vi "Access DB Path.vi"(9 "Password":string, 10 "ping":bool, 11 "database":string="database1.mdb") -> (2 "Connection information":string, 3 "Path out":string)   [LabVIEW 2016, in "Access Lib.lvlib"]
uses:
  Access Lib.lvlib
  <vilib>/Utility/sysdir.llb/System Directory Type.ctl
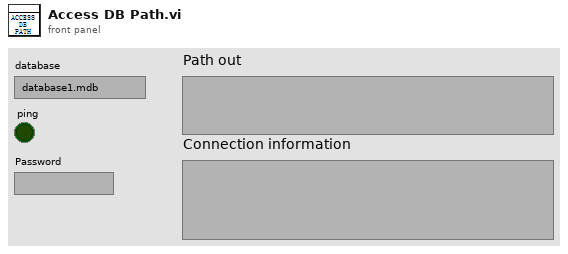
[diagram p1: front panel]
types:
  T1 = typedef "System Directory Type.ctl" = i32
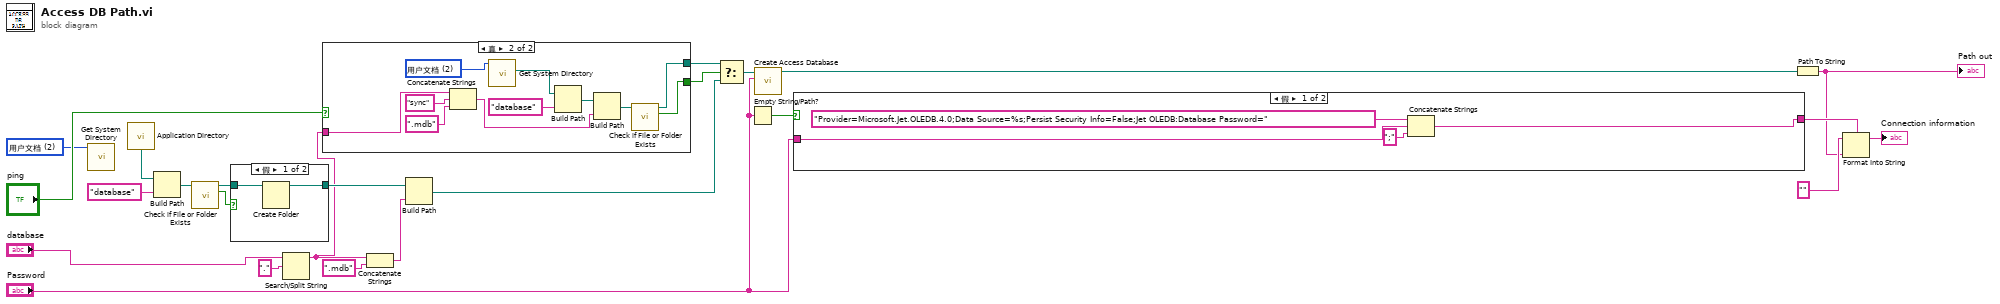
[diagram p0: block diagram]
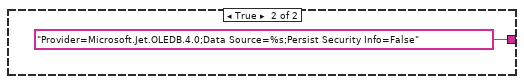
[diagram p3: hidden frame]
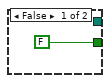
[diagram p4: hidden frame]
diagram:
  w10 = T1 2 items=["用户目录"=0, "用户桌面"=1, "用户文档"=2, "用户应用程序数据"=3, "用户设置"=4, "用户临时目录"=5, "公共文档"=6, "公共应用程序数据"=7, "公共设置"=8, "公共缓存"=13, "系统核心库"=9, "系统安装库"=10, "应用程序文件"=11, "启动盘根目录"=12] ("system directory type")
  n1 = call <vilib>:"Get System Directory.vi"("system directory type"=w10) -> ()  [unwired: 10 in, 1 out]
  n2 = call <vilib>:"Application Directory.vi"() -> ("Application Directory"=w1:path)
  n3 = Build Path(base path=w1, name or relative path="database" ("名称或相对路径")) -> (appended path=w8:path)
  n4 = call <vilib>:"Check if File or Folder Exists.vi"("path"=w8) -> ("file or folder exists?"=w13:bool, "dup path"=w12:path)  [unwired: 8 in, 1 out]
  n5 = case shown="假" w13 {
    tunnel: w12 -> [w26 w27]
    tunnel: [w25 w27] -> w11
    frame False {
      n6 = Create Folder(path (use dialog)=w26) -> (created path=w25:path)  [unwired: 2 in, 2 out]
    }
    frame True {
    }
  }
  n7 = Search/Split String(string="database", search string/char (-)="." ("搜索字符串/字符(-)")) -> (substring before match=w2:string)  [unwired: 1 in, 2 out]
  n8 = case shown="真" "ping" {
    tunnel: [FALSE ("file or folder exists?") w34] -> w7
    tunnel: [_ w33] -> w6
    tunnel: w2 -> [_ w29]
    frame False {
    }
    frame True {
      w39 = T1 2 items=["用户目录"=0, "用户桌面"=1, "用户文档"=2, "用户应用程序数据"=3, "用户设置"=4, "用户临时目录"=5, "公共文档"=6, "公共应用程序数据"=7, "公共设置"=8, "公共缓存"=13, "系统核心库"=9, "系统安装库"=10, "应用程序文件"=11, "启动盘根目录"=12] ("system directory type")
      n9 = Concatenate Strings(w29, "sync" ("字符串"), ".mdb" ("字符串")) -> (w30:string)
      n10 = call <vilib>:"Get System Directory.vi"("system directory type"=w39) -> ("system directory"=w38:path)  [unwired: 10 in]
      n11 = Build Path(base path=w38, name or relative path="database" ("名称或相对路径")) -> (appended path=w36:path)
      n12 = Build Path(base path=w36, name or relative path=w30) -> (appended path=w35:path)
      n13 = call <vilib>:"Check if File or Folder Exists.vi"("path"=w35) -> ("file or folder exists?"=w34:bool, "dup path"=w33:path)  [unwired: 8 in, 1 out]
    }
  }
  n14 = Concatenate Strings(w2, ".mdb" ("字符串")) -> (w3:string)
  n15 = Build Path(base path=w11, name or relative path=w3) -> (appended path=w5:path)
  n16 = Select(t=w6, s=w7, f=w5) -> (s? t:f=w4:path)
  n17 = Empty String/Path?(string/path="Password") -> (empty?=w22:bool)
  n18 = call "Create Access Database.vi"("Password"="Password", "路径"=w4) -> ("路径 out"=w23:path)  [unwired: 8 in, 1 out]
  n19 = case shown="假" w22 {
    tunnel: [w40 "Provider=Microsoft.Jet.OLEDB.4.0;Data Source=%s;Persist Security Info=False" ("格式字符串")] -> w20
    tunnel: "Password" -> [w43 _]
    frame False {
      n20 = Concatenate Strings("Provider=Microsoft.Jet.OLEDB.4.0;Data Source=%s;Persist Security Info=False;Jet OLEDB:Database Password=" ("格式字符串"), w43, ";" ("字符串")) -> (w40:string)
    }
    frame True {
    }
  }
  n21 = Path To String(path=w23) -> (string=w18:string)
  "Path out" <- w18
  n22 = Format Into String(format string=w20, initial string="" ("初始字符串"), w18) -> (resulting string=→"Connection information":string)  [unwired: 1 in, 1 out]
